vi "FTW-JSON-Reflection-Type.vi"(5 "JSON String":string, 9 "Starting Offset":i32, 11 "error in":errorcluster) -> (4 "Data Name":string, 6 "Element":string, 8 "JSON Type":T1, 10 "Offset after Match":i32, 15 "error out":errorcluster)   [LabVIEW 2015]
uses:
  FTW-JSON-Type.ctl
panel:
  out "Found Match?":bool
  # "Inputs"
  # "Outputs"
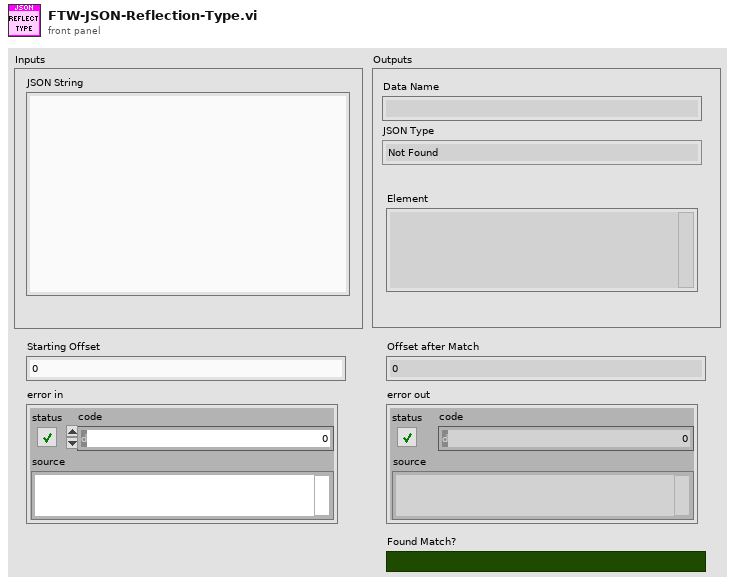
[diagram p1: front panel]
types:
  T1 = typedef "FTW-JSON-Type.ctl" = enum8{"Not Found", "Object", "Array", "String", "Number", "Boolean", "null"}
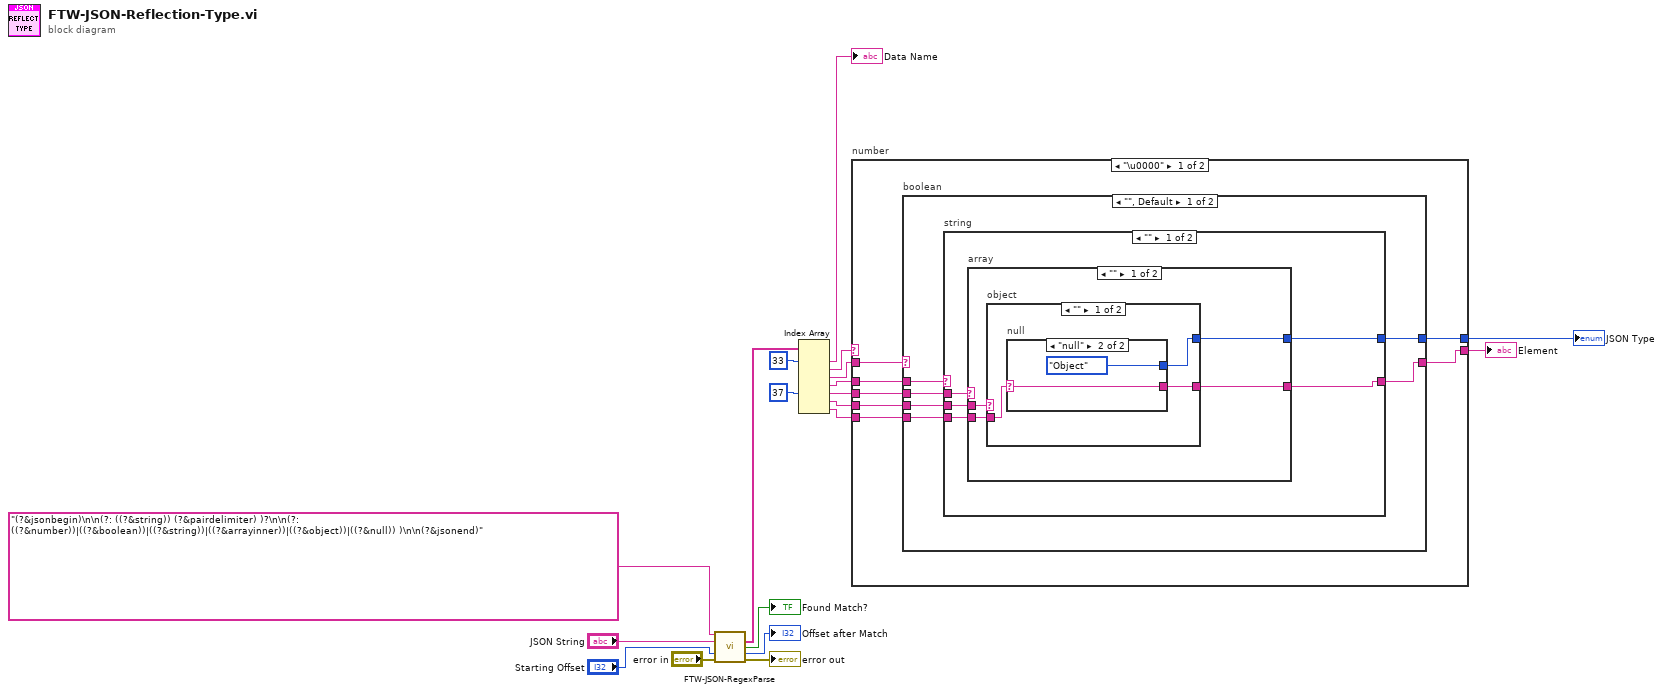
[diagram p0: block diagram]
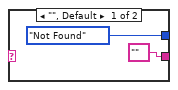
[diagram p2: hidden frame]
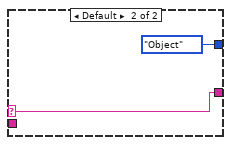
[diagram p3: hidden frame]
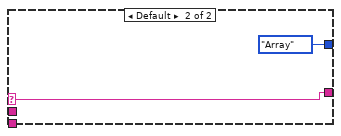
[diagram p4: hidden frame]
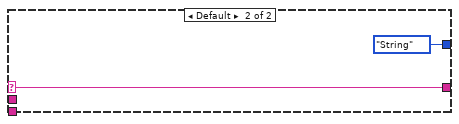
[diagram p5: hidden frame]
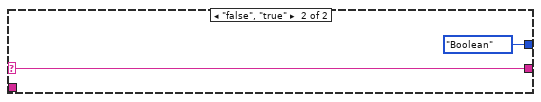
[diagram p6: hidden frame]
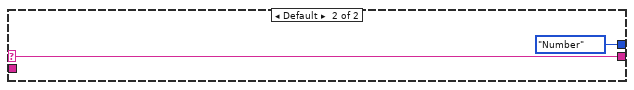
[diagram p7: hidden frame]
diagram:
  n1 = call "FTW-JSON-RegexParse.vi"("Regular Expression using JSON subroutines"="(?&jsonbegin)\n\n(?: ((?&string)) (?&pairdelimiter) )?\n\n(?: ((?&number))|((?&boolean))|((?&string))|((?&arrayinner))|((?&object))|((?&null)) )\n\n(?&jsonend)", "Input String"="JSON String", "Starting Offset"="Starting Offset", "error in"="error in") -> ("Submatches"=w19:string[], "Found Match?"=→"Found Match?":bool, "Offset after Match"=→"Offset after Match":i32, "error out"=→"error out":errorcluster)  [unwired: 7 in, 1 out]
  n2 = Index Array(array=w19, index #1=33 ("index"), index #5=37 ("index")) -> (element #1=→"Data Name":string, element #2=w11:string, element #3=w9:string, element #4=w7:string, element #5=w6:string, element #6=w5:string, element #7=w4:string)  [unwired: 5 in]
  n3 = case "number" shown="\"\"" w11 {
    selector: w11 -> [_ w57]
    tunnel: [w26 FTW-JSON-Type."Number" ("JSON Type")] -> w10
    tunnel: w9 -> [w25 _]
    tunnel: [w24 w57] -> w8
    tunnel: w7 -> [w23 _]
    tunnel: w6 -> [w22 _]
    tunnel: w5 -> [w21 _]
    tunnel: w4 -> [w20 _]
    frame "\u0000" {
      n4 = case "boolean" shown="\"\", Default" w25 {
        selector: w25 -> [_ w55]
        tunnel: [w32 FTW-JSON-Type."Boolean" ("JSON Type")] -> w26
        tunnel: [w30 w55] -> w24
        tunnel: w23 -> [w31 _]
        tunnel: w22 -> [w29 _]
        tunnel: w21 -> [w28 _]
        tunnel: w20 -> [w27 _]
        frame "", Default {
          n5 = case "string" shown="\"\"" w31 {
            selector: w31 -> [_ w53]
            tunnel: [w36 FTW-JSON-Type."String" ("JSON Type")] -> w32
            tunnel: [w35 w53] -> w30
            tunnel: w29 -> [w37 _]
            tunnel: w28 -> [w34 _]
            tunnel: w27 -> [w33 _]
            frame "" {
              n6 = case "array" shown="\"\"" w37 {
                selector: w37 -> [_ w51]
                tunnel: [w41 FTW-JSON-Type."Array" ("JSON Type")] -> w36
                tunnel: [w40 w51] -> w35
                tunnel: w34 -> [w39 _]
                tunnel: w33 -> [w38 _]
                frame "" {
                  n7 = case "object" shown="\"\"" w39 {
                    selector: w39 -> [_ w49]
                    tunnel: [w43 FTW-JSON-Type."Object" ("JSON Type")] -> w41
                    tunnel: [w44 w49] -> w40
                    tunnel: w38 -> [w42 _]
                    frame "" {
                      n8 = case "null" shown="\"null\"" w42 {
                        selector: w42 -> [_ w47]
                        tunnel: [FTW-JSON-Type."Not Found" ("JSON Type") FTW-JSON-Type."Object" ("JSON Type")] -> w43
                        tunnel: ["" w47] -> w44
                        frame "", Default {
                        }
                        frame "null" {
                        }
                      }
                    }
                    frame Default {
                    }
                  }
                }
                frame Default {
                }
              }
            }
            frame Default {
            }
          }
        }
        frame "false", "true" {
        }
      }
    }
    frame Default {
    }
  }
  "JSON Type" <- w10
  "Element" <- w8
